vi "Test Add New State.vi"(8 "error in (no error)":errorcluster) -> (0 "error out":errorcluster)   [LabVIEW 2013, in "TEST JKI State Machine API.lvlib"]
uses:
  TEST JKI State Machine API.lvlib
  <vilib>/addons/_JKI Toolkits/Caraya/classes/Assert/Assert.lvclass
  <vilib>/addons/_JKI Toolkits/Caraya/classes/Test/Test.lvclass
  source/JKI SM/JKI SM.lvclass
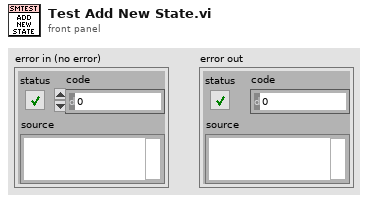
[diagram p1: front panel]
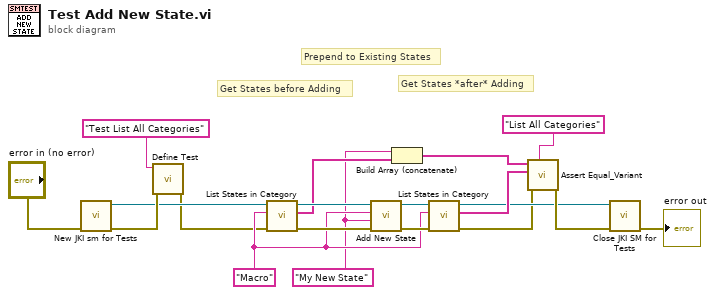
[diagram p0: block diagram]
diagram:
  w1 = "My New State" ("State Name")
  w8 = "Macro" ("Category")
  # "Get States *after* Adding"
  # "Get States before Adding"
  # "Prepend to Existing States"
  n1 = call "New JKI sm for Tests.vi"("error in (no error)"="error in (no error)") -> ("error out"=w19:errorcluster, "JKI SM out"=w13:refnum<class "JKI SM.lvclass">)  [unwired: 9 in]
  n2 = call <vilib>:"Define Test.vi"("error in (no error)"=w19, "Label (VI Title)"="Test List All Categories") -> ("error out"=w3:errorcluster)  [unwired: 9 in]
  n3 = call "List States in Category.vi"("error in (no error)"=w3, "Category"=w8, "JKI SM in"=w13) -> ("error out"=w11:errorcluster, "States"=w7:string[], "JKI SM out"=w12:refnum<class "JKI SM.lvclass">)  [unwired: 4 in, 2 out]
  n4 = call "Add New State.vi"("error in (no error)"=w11, "State Name"=w1, "Category (Optional)"=w8, "JKI SM in"=w12) -> ("error out"=w9:errorcluster, "JKI SM out"=w10:refnum<class "JKI SM.lvclass">)  [unwired: 5 in, 1 out]
  n5 = Build Array (concatenate)(w1, w7) -> (w6:string[])
  n6 = call "List States in Category.vi"("error in (no error)"=w9, "Category"=w8, "JKI SM in"=w10) -> ("error out"=w2:errorcluster, "States"=w5:string[], "JKI SM out"=w4:refnum<class "JKI SM.lvclass">)  [unwired: 4 in, 2 out]
  n7 = call <vilib>:"Assert Equal_Variant.vi"("Label"="List All Categories", "error in (no error)"=w2, "Y"=w5, "X"=w6) -> ("error out"=w16:errorcluster)  [unwired: 7 in]
  n8 = call "Close JKI SM for Tests.vi"("error in (no error)"=w16, "JKI SM in"=w4) -> ("error out"=→"error out":errorcluster)  [unwired: 9 in]
